vi "Read Introspection Output.vi"(8 "error in (no error)":errorcluster, 11 "ONNX Class in":refnum<class "ONNX Class.lvclass">) -> (0 "error out":errorcluster, 2 "Introspection":T1, 3 "ONNX Class out":refnum<class "ONNX Class.lvclass">)   [LabVIEW 2017, in "ONNX Class Library.lvlib" / "ONNX Class.lvclass"]
uses:
  ONNX Class.lvclass
  ONNX Class.lvclass/ONNX Class.ctl
  TypeDef/IO.ctl
  ONNX Class Library.lvlib
  TypeDef/Introspection.ctl
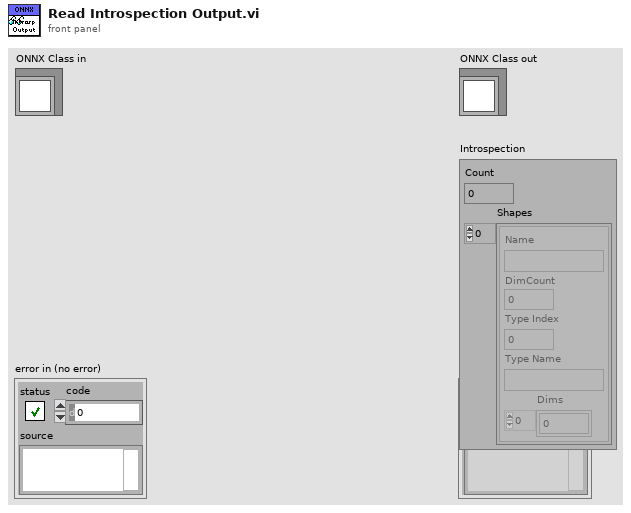
[diagram p1: front panel]
types:
  T1 = typedef "ONNX Class Library.lvlib/Introspection.ctl" = cluster{"Count":i32, "Shapes":T2[]}
  T2 = typedef "ONNX Class Library.lvlib/IO.ctl" = cluster{"Name":string, "DimCount":i32, "Type Index":i32, "Type Name":string, "Dims":i64[]}
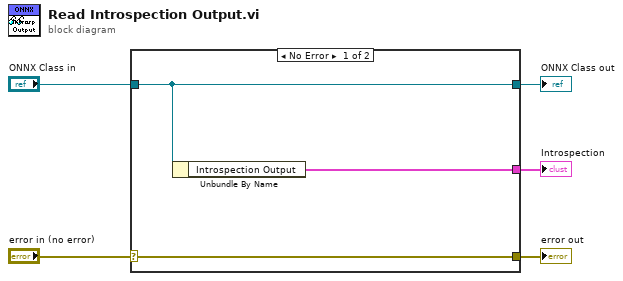
[diagram p0: block diagram]
diagram:
  n1 = case shown="No Error" "error in (no error)" {
    selector: "error in (no error)" -> [w8 w9]
    tunnel: [w8 w9] -> w4
    tunnel: [w7 w10] -> w2
    tunnel: "ONNX Class in" -> [w7 w10]
    tunnel: [w6 _] -> w1
    frame No Error {
      n2 = Unbundle By Name(w7) -> ("Introspection Output"=w6:T1)
    }
    frame Error {
    }
  }
  "error out" <- w4
  "ONNX Class out" <- w2
  "Introspection" <- w1
